vi "PCU_Sample.vi"() -> ()   [LabVIEW 2017]
uses:
  D:/test/FULLband-sts/Fullband_Sample/DLL/InstrumentDLL.dll
  DLL/InstrumentDLL.dll
panel:
  out "PCU":refnum<k24>
  out "LAN Port number":i32
  in  "Btn_GetLAN_Port":bool
  out "IP Address":string
  in  "Btn_GetIPAddress":bool
  in  "btnGet_Range":bool
  out "txtcurrentrange":string
  in  "btnAdjust_Range":bool
  in  "btnSet_SOP":bool
  in  "SOP Stauts":u16(ring)
  out "Serial number":string
  out "Product":string
  out "F/ W Vesion":string
  out "Wavelength range":string
  out "PCU-100 Control ID":string
  in  "Port number":i32
  in  "Target":enum32{"rdo100", "rdo110"}(radio)
  in  "Communication":T1(radio)
  in  "Terminator":enum32{"Cr", "Lf", "CrLf"}(radio)
  in  "Btn_Connect":bool
  in  "Btn_DisConnect":bool
  in  "Address/Device number":string
  in  "btnControl_ID":bool
  in  "PCU-100 Control ID":enum16{""}(ring)
  in  "Usb resouce":enum16{""}(ring)
  in  "btnUsb_resouce":bool
  in  "USB device number":string
  in  "btnSplit":bool
  out "GPIB Address":dbl
  out "GPIB Boad":dbl
  in  "btnGet_Visa":bool
  in  "Visa String":u16(ring) items=["GPIB0::5::INSTR"]
  # "0. Connect Tool"
  # "1. Connect"
  # "Information"
  # "2.Function"
  # "Power Control"
  # "SOP Control"
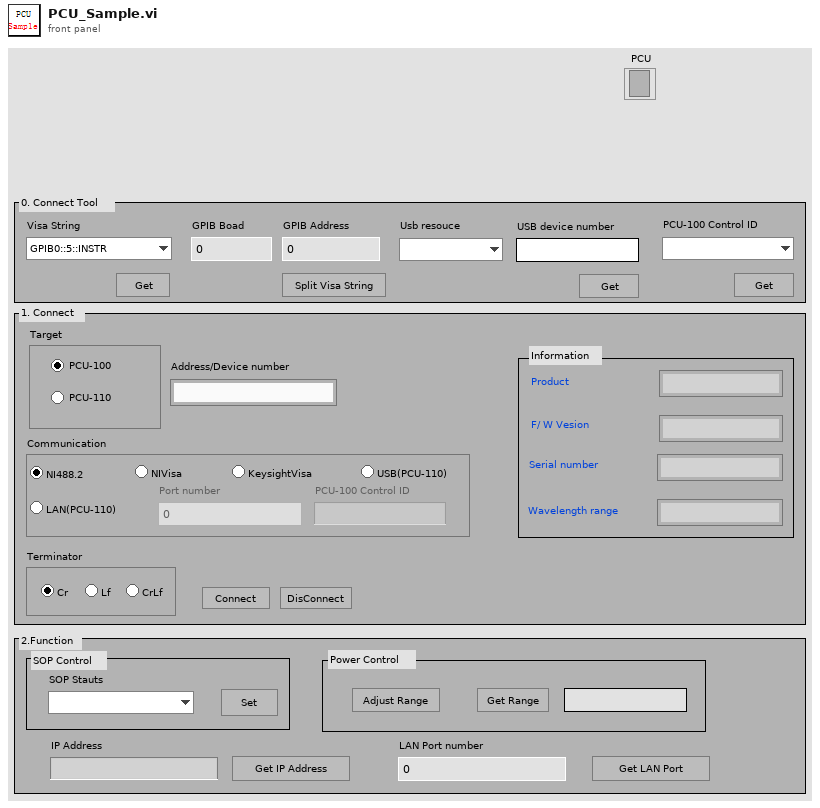
[diagram p1: front panel]
types:
  T1 = enum32{"rdiNI488", "rdiNIvisa", "rdikeysightvisa", "rdiUSB", "rdiLAN"}
  T2 = enum8{"Enabled", "Disabled", "Disabled and Grayed Out"}
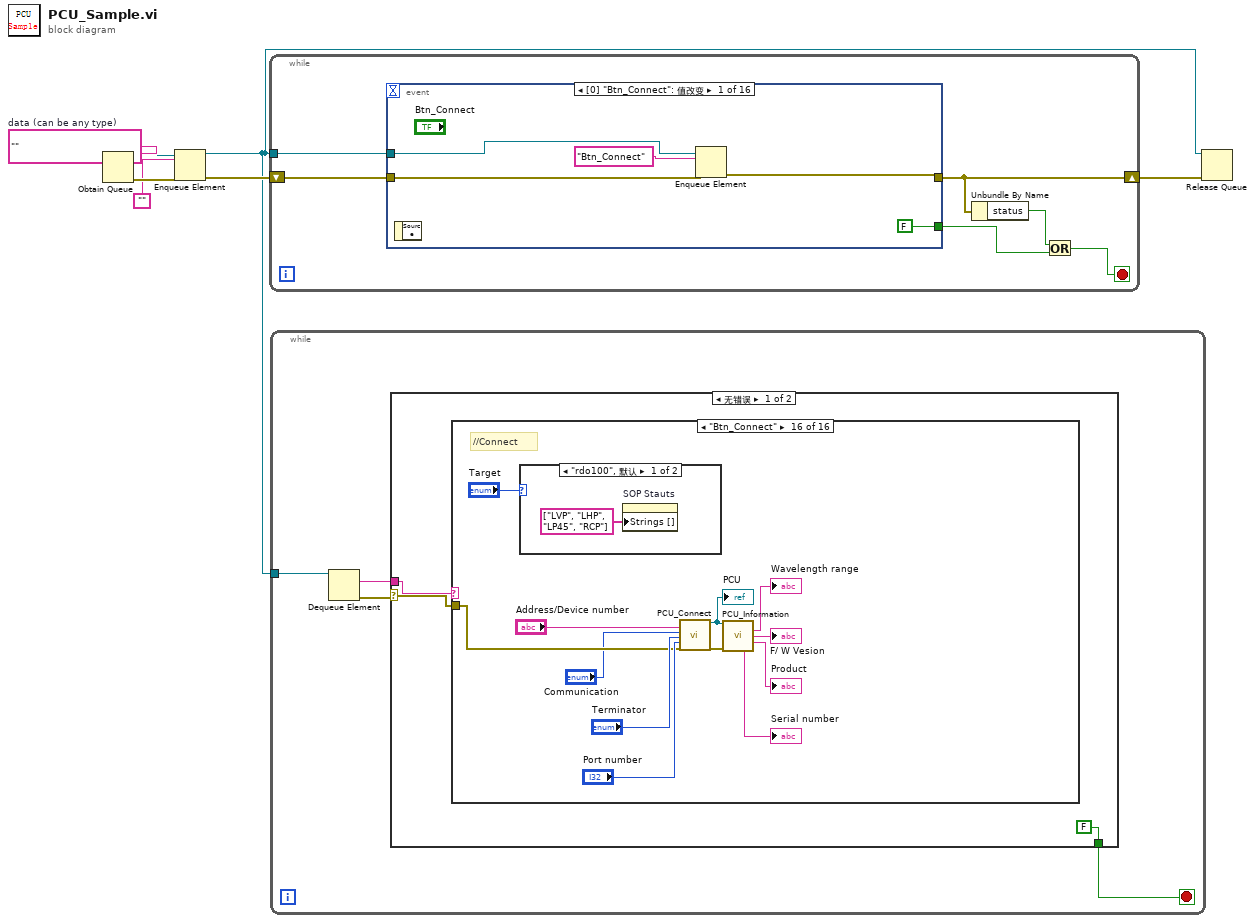
[diagram p0: block diagram]
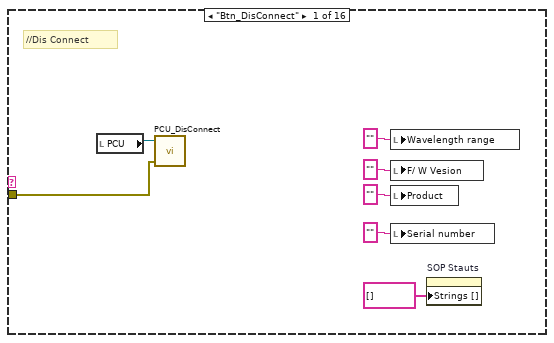
[diagram p2: hidden frame]
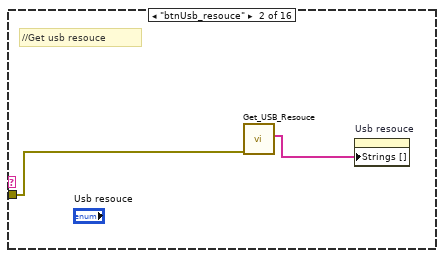
[diagram p3: hidden frame]
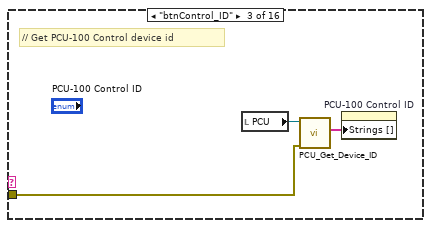
[diagram p4: hidden frame]
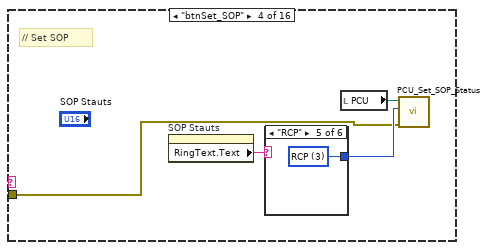
[diagram p5: hidden frame]
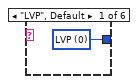
[diagram p6: hidden frame]
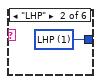
[diagram p7: hidden frame]
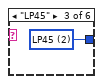
[diagram p8: hidden frame]
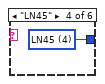
[diagram p9: hidden frame]
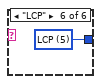
[diagram p10: hidden frame]
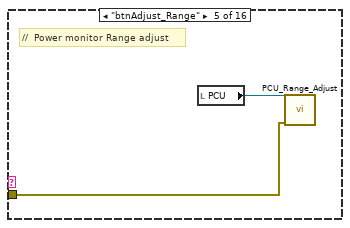
[diagram p11: hidden frame]
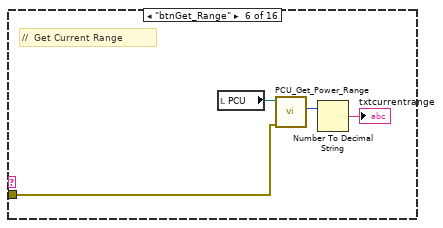
[diagram p12: hidden frame]
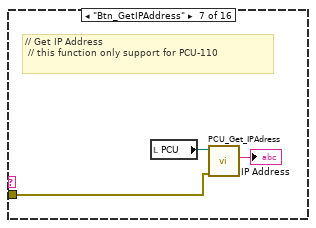
[diagram p13: hidden frame]
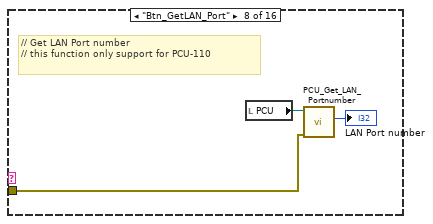
[diagram p14: hidden frame]
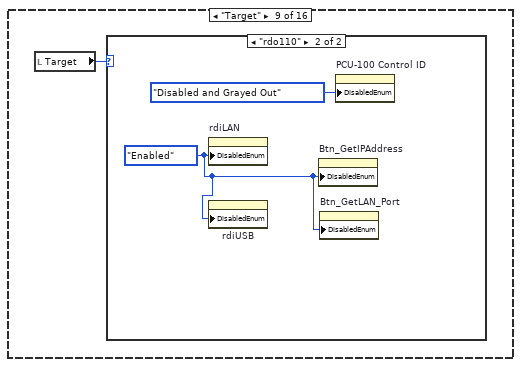
[diagram p15: hidden frame]
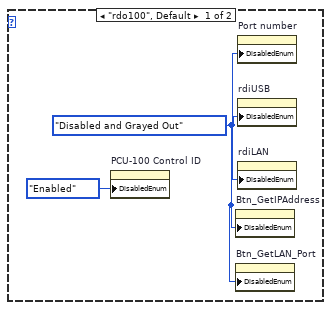
[diagram p16: hidden frame]
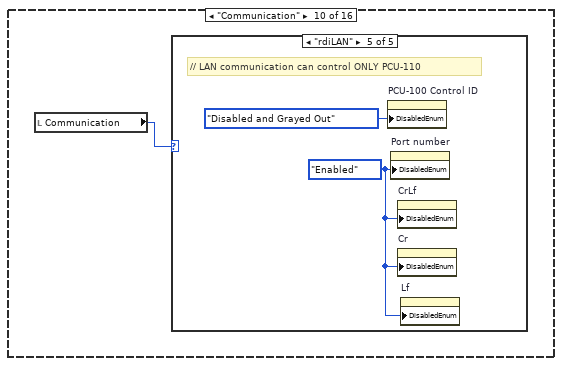
[diagram p17: hidden frame]
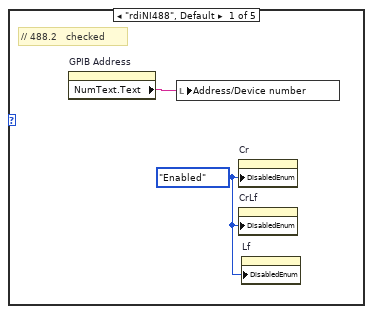
[diagram p18: hidden frame]
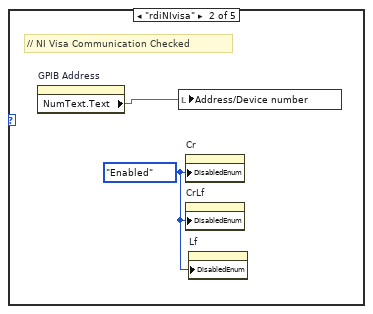
[diagram p19: hidden frame]
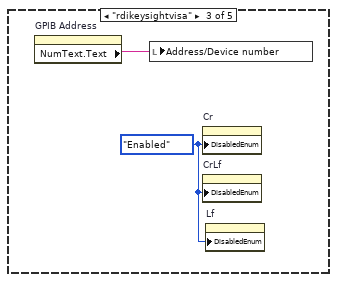
[diagram p20: hidden frame]
diagram:
  w6 = ""  # data (can be any type)
  n1 = Obtain Queue(element data type=w6) -> (queue out=w5:refnum<queue>, error out=w7:errorcluster)  [unwired: 4 in, 1 out]
  n2 = Enqueue Element(queue=w5, element="", error in (no error)=w7) -> (queue out=w1:refnum<queue>, error out=w3:errorcluster)  [unwired: 1 in, 1 out]
  n3 = while {
    tunnel: w1 -> [w12]
    shift-right: [w9] -> w2
    shift-left: w3 -> [w13]
    stop <- w10 stop-if-true
    n4 = event shown="[0] \"Btn_Connect\": 值改变" {
      selector: _ -> [_ _ _ _ _ _ _ _ _ _ _ _ _ _ _ _]
      dyn-events: _ -> [_ _ _ _ _ _ _ _ _ _ _ _ _ _ _ _]
      timeout: _ -> [_ _ _ _ _ _ _ _ _ _ _ _ _ _ _ _]
      tunnel: w13 -> [w16 w21 w26 w30 w34 w38 w42 w46 w50 w54 w58 w62 w66 w70 w74 _]
      tunnel: w12 -> [w17 w22 w25 w29 w33 w37 w41 w45 w49 w53 w57 w61 w65 w69 w73 _]
      tunnel: [w15 w20 w24 w28 w32 w36 w40 w44 w48 w52 w56 w60 w64 w68 w72 _] -> w9
      tunnel: [FALSE ("stop") FALSE ("stop") _ _ _ _ _ _ _ _ _ _ _ _ _ TRUE ("stop")] -> w8
      event "Btn_Connect": Value Change {
        n5 = event-data() -> ()  [unwired: 1 in, 1 out]
        n6 = Enqueue Element(queue=w17, element="Btn_Connect" ("元素"), error in (no error)=w16) -> (error out=w15:errorcluster)  [unwired: 1 in, 2 out]
      }
      event "Btn_DisConnect": Value Change {
        n7 = event-data() -> ()  [unwired: 1 in, 1 out]
        n8 = Enqueue Element(queue=w22, element="Btn_DisConnect" ("元素"), error in (no error)=w21) -> (error out=w20:errorcluster)  [unwired: 1 in, 2 out]
      }
      event "btnGet_Visa": Value Change {
        n9 = event-data() -> ()  [unwired: 1 in, 1 out]
        n10 = Enqueue Element(queue=w25, element="btnGet_Visa" ("元素"), error in (no error)=w26) -> (error out=w24:errorcluster)  [unwired: 1 in, 2 out]
      }
      event "btnSplit": Value Change {
        n11 = event-data() -> ()  [unwired: 1 in, 1 out]
        n12 = Enqueue Element(queue=w29, element="btnSplit" ("元素"), error in (no error)=w30) -> (error out=w28:errorcluster)  [unwired: 1 in, 2 out]
      }
      event "btnUsb_resouce": Value Change {
        n13 = event-data() -> ()  [unwired: 1 in, 1 out]
        n14 = Enqueue Element(queue=w33, element="btnUsb_resouce" ("元素"), error in (no error)=w34) -> (error out=w32:errorcluster)  [unwired: 1 in, 2 out]
      }
      event "btnControl_ID": Value Change {
        n15 = event-data() -> ()  [unwired: 1 in, 1 out]
        n16 = Enqueue Element(queue=w37, element="btnControl_ID" ("元素"), error in (no error)=w38) -> (error out=w36:errorcluster)  [unwired: 1 in, 2 out]
      }
      event "btnSet_SOP": Value Change {
        n17 = event-data() -> ()  [unwired: 1 in, 1 out]
        n18 = Enqueue Element(queue=w41, element="btnSet_SOP" ("元素"), error in (no error)=w42) -> (error out=w40:errorcluster)  [unwired: 1 in, 2 out]
      }
      event "btnAdjust_Range": Value Change {
        n19 = event-data() -> ()  [unwired: 1 in, 1 out]
        n20 = Enqueue Element(queue=w45, element="btnAdjust_Range" ("元素"), error in (no error)=w46) -> (error out=w44:errorcluster)  [unwired: 1 in, 2 out]
      }
      event "btnGet_Range": Value Change {
        n21 = event-data() -> ()  [unwired: 1 in, 1 out]
        n22 = Enqueue Element(queue=w49, element="btnGet_Range" ("元素"), error in (no error)=w50) -> (error out=w48:errorcluster)  [unwired: 1 in, 2 out]
      }
      event "Btn_GetIPAddress": Value Change {
        n23 = event-data() -> ()  [unwired: 1 in, 1 out]
        n24 = Enqueue Element(queue=w53, element="Btn_GetIPAddress" ("元素"), error in (no error)=w54) -> (error out=w52:errorcluster)  [unwired: 1 in, 2 out]
      }
      event "Btn_GetLAN_Port": Value Change {
        n25 = event-data() -> ()  [unwired: 1 in, 1 out]
        n26 = Enqueue Element(queue=w57, element="Btn_GetLAN_Port" ("元素"), error in (no error)=w58) -> (error out=w56:errorcluster)  [unwired: 1 in, 2 out]
      }
      event "Target": Value Change {
        n27 = event-data() -> ()  [unwired: 1 in, 1 out]
        n28 = Enqueue Element(queue=w61, element="Target" ("元素"), error in (no error)=w62) -> (error out=w60:errorcluster)  [unwired: 1 in, 2 out]
      }
      event "Communication": Value Change {
        n29 = event-data() -> ()  [unwired: 1 in, 1 out]
        n30 = Enqueue Element(queue=w65, element="Communication" ("元素"), error in (no error)=w66) -> (error out=w64:errorcluster)  [unwired: 1 in, 2 out]
      }
      event "Usb resouce": Value Change {
        n31 = event-data() -> ()  [unwired: 1 in, 1 out]
        n32 = Enqueue Element(queue=w69, element="Usb resouce" ("元素"), error in (no error)=w70) -> (error out=w68:errorcluster)  [unwired: 1 in, 2 out]
      }
      event "PCU-100 Control ID": Value Change {
        n33 = event-data() -> ()  [unwired: 1 in, 1 out]
        n34 = Enqueue Element(queue=w73, element="PCU-100 Control ID" ("元素"), error in (no error)=w74) -> (error out=w72:errorcluster)  [unwired: 1 in, 2 out]
      }
      event Panel Close {
        n35 = event-data() -> ()  [unwired: 1 in, 1 out]
      }
    }
    n36 = Unbundle By Name(w9) -> ("status"=w11:bool)
    n37 = Or(x=w11, y=w8) -> (x .or. y?=w10:bool)
  }
  n38 = while {
    tunnel: w1 -> [w79]
    stop <- w77 stop-if-true
    n39 = Dequeue Element(queue=w79) -> (element=w78:string, error out=w80:errorcluster)  [unwired: 2 in, 2 out]
    n40 = case shown="无错误" w80 {
      selector: w80 -> [w81 _]
      tunnel: w78 -> [w83 _]
      tunnel: [FALSE TRUE] -> w77
      frame No Error {
        n41 = case shown="\"Btn_Connect\"" w83 {
          tunnel: w81 -> [w84 w91 w93 w96 w106 w108 w112 w115 _ _ _ _ _ w139 _ w163]
          frame "Btn_DisConnect" {
            # "//Dis Connect"
            n42 = local read "PCU"() -> (w85:refnum<k24>)
            n43 = call "PCU_DisConnect.vi"("error in (no error)"=w84, ".NET Reference in"=w85) -> ()  [unwired: 2 in, 2 out]
            n44 = local write "Wavelength range"("" ("Wavelength range")) -> ()
            n45 = local write "F/ W Vesion"("" ("F/ W Vesion")) -> ()
            n46 = local write "Product"("" ("Product")) -> ()
            n47 = local write "Serial number"("" ("Serial number")) -> ()
            n48 = property on="SOP Stauts" class="Ring (严格)"("Strings []"=string[] [] ("字符串[]")) -> ()  [unwired: 2 in, 2 out]
          }
          frame "btnUsb_resouce" {
            # "//Get usb resouce"
            n49 = call "Get_USB_Resouce.vi"("error in (no error)"=w91) -> ("Get_USB_Resouce"=w92:string[])  [unwired: 8 in, 2 out]
            n50 = property on="Usb resouce" class="Enum (严格)"("Strings []"=w92) -> ()  [unwired: 2 in, 2 out]
          }
          frame "btnControl_ID" {
            # "// Get PCU-100 Control device id"
            n51 = local read "PCU"() -> (w95:refnum<k24>)
            n52 = call "PCU_Get_Device_ID.vi"("error in (no error)"=w93, ".NET Reference in"=w95) -> ("id"=w94:string[])  [unwired: 7 in, 2 out]
            n53 = property on="PCU-100 Control ID" class="Enum (严格)"("Strings []"=w94) -> ()  [unwired: 2 in, 2 out]
          }
          frame "btnSet_SOP" {
            # "// Set SOP"
            n54 = property on="SOP Stauts" class="Ring (严格)"() -> ("RingText.Text"=w98:string)  [unwired: 2 in, 2 out]
            n55 = case shown="\"RCP\"" w98 {
              tunnel: [w100 w101 w102 w103 w104 w105] -> w97
              frame "LVP", Default {
                w100 = 0 items=["LVP", "LHP", "LP45", "RCP", "LN45", "LCP"] ("status")
              }
              frame "LHP" {
                w101 = 1 items=["LVP", "LHP", "LP45", "RCP", "LN45", "LCP"] ("status")
              }
              frame "LP45" {
                w102 = 2 items=["LVP", "LHP", "LP45", "RCP", "LN45", "LCP"] ("status")
              }
              frame "LN45" {
                w103 = 4 items=["LVP", "LHP", "LP45", "RCP", "LN45", "LCP"] ("status")
              }
              frame "RCP" {
                w104 = 3 items=["LVP", "LHP", "LP45", "RCP", "LN45", "LCP"] ("status")
              }
              frame "LCP" {
                w105 = 5 items=["LVP", "LHP", "LP45", "RCP", "LN45", "LCP"] ("status")
              }
            }
            n56 = local read "PCU"() -> (w99:refnum<k24>)
            n57 = call "PCU_Set_SOP_Status.vi"("error in (no error)"=w96, "status"=w97, ".NET Reference in"=w99) -> ()  [unwired: 7 in, 2 out]
          }
          frame "btnAdjust_Range" {
            # "//  Power monitor Range adjust"
            n58 = local read "PCU"() -> (w107:refnum<k24>)
            n59 = call "PCU_Range_Adjust.vi"("error in (no error)"=w106, ".NET Reference in"=w107) -> ()  [unwired: 8 in, 2 out]
          }
          frame "btnGet_Range" {
            # "//  Get Current Range"
            n60 = local read "PCU"() -> (w111:refnum<k24>)
            n61 = call "PCU_Get_Power_Range.vi"("error in (no error)"=w108, ".NET Reference in"=w111) -> ("range"=w109:i32)  [unwired: 7 in, 2 out]
            n62 = Number To Decimal String(number=w109) -> (decimal integer string=→"txtcurrentrange":string)  [unwired: 1 in]
          }
          frame "Btn_GetIPAddress" {
            # "// Get IP Address\n // this function only support for PCU-110"
            n63 = local read "PCU"() -> (w114:refnum<k24>)
            n64 = call "PCU_Get_IPAdress.vi"("error in (no error)"=w112, ".NET Reference in"=w114) -> ("address"=→"IP Address":string)  [unwired: 7 in, 2 out]
          }
          frame "Btn_GetLAN_Port" {
            # "// Get LAN Port number\n// this function only support for PCU-110"
            n65 = local read "PCU"() -> (w117:refnum<k24>)
            n66 = call "PCU_Get_LAN_Portnumber.vi"("error in (no error)"=w115, ".NET Reference in"=w117) -> ("port"=→"LAN Port number":i32)  [unwired: 7 in, 2 out]
          }
          frame "Target" {
            n67 = local read "Target"() -> (w118:enum32{"rdo100", "rdo110"})
            n68 = case shown="\"rdo110\"" w118 {
              frame "rdo100", Default {
                w119 = T2."Disabled and Grayed Out" ("禁用")
                n69 = property on="PCU-100 Control ID" class="Str"("DisabledEnum"=T2."Enabled" ("禁用")) -> ()  [unwired: 2 in, 2 out]
                n70 = property on="Btn_GetIPAddress" class="Bool"("DisabledEnum"=w119) -> ()  [unwired: 2 in, 2 out]
                n71 = property on="Btn_GetLAN_Port" class="Bool"("DisabledEnum"=w119) -> ()  [unwired: 2 in, 2 out]
                n72 = property on="Port number" class="DigNum (严格)"("DisabledEnum"=w119) -> ()  [unwired: 2 in, 2 out]
                n73 = property on="rdiUSB" class="Bool (严格)"("DisabledEnum"=w119) -> ()  [unwired: 2 in, 2 out]
                n74 = property on="rdiLAN" class="Bool (严格)"("DisabledEnum"=w119) -> ()  [unwired: 2 in, 2 out]
              }
              frame "rdo110" {
                w121 = T2."Enabled" ("禁用")
                n75 = property on="rdiLAN" class="Bool (严格)"("DisabledEnum"=w121) -> ()  [unwired: 2 in, 2 out]
                n76 = property on="rdiUSB" class="Bool (严格)"("DisabledEnum"=w121) -> ()  [unwired: 2 in, 2 out]
                n77 = property on="Btn_GetIPAddress" class="Bool"("DisabledEnum"=w121) -> ()  [unwired: 2 in, 2 out]
                n78 = property on="Btn_GetLAN_Port" class="Bool"("DisabledEnum"=w121) -> ()  [unwired: 2 in, 2 out]
                n79 = property on="PCU-100 Control ID" class="Str"("DisabledEnum"=T2."Disabled and Grayed Out" ("禁用")) -> ()  [unwired: 2 in, 2 out]
              }
            }
          }
          frame "Communication" {
            n80 = local read "Communication"() -> (w123:T1)
            n81 = case shown="\"rdiLAN\"" w123 {
              frame "rdiNI488", Default {
                w125 = T2."Enabled" ("禁用")
                # "// 488.2　checked"
                n82 = property on="GPIB Address" class="DigNum (严格)"() -> ("NumText.Text"=w124:string)  [unwired: 2 in, 2 out]
                n83 = local write "Address/Device number"(w124) -> ()
                n84 = property on="Cr" class="Bool (严格)"("DisabledEnum"=w125) -> ()  [unwired: 2 in, 2 out]
                n85 = property on="CrLf" class="Bool (严格)"("DisabledEnum"=w125) -> ()  [unwired: 2 in, 2 out]
                n86 = property on="Lf" class="Bool (严格)"("DisabledEnum"=w125) -> ()  [unwired: 2 in, 2 out]
              }
              frame "rdiNIvisa" {
                w127 = T2."Enabled" ("禁用")
                # "// NI Visa Communication Checked"
                n87 = property on="GPIB Address" class="DigNum (严格)"() -> ("NumText.Text"=w126:string)  [unwired: 2 in, 2 out]
                n88 = local write "Address/Device number"(w126) -> ()
                n89 = property on="Cr" class="Bool (严格)"("DisabledEnum"=w127) -> ()  [unwired: 2 in, 2 out]
                n90 = property on="CrLf" class="Bool (严格)"("DisabledEnum"=w127) -> ()  [unwired: 2 in, 2 out]
                n91 = property on="Lf" class="Bool (严格)"("DisabledEnum"=w127) -> ()  [unwired: 2 in, 2 out]
              }
              frame "rdikeysightvisa" {
                w129 = T2."Enabled" ("禁用")
                n92 = property on="GPIB Address" class="DigNum (严格)"() -> ("NumText.Text"=w128:string)  [unwired: 2 in, 2 out]
                n93 = local write "Address/Device number"(w128) -> ()
                n94 = property on="Cr" class="Bool (严格)"("DisabledEnum"=w129) -> ()  [unwired: 2 in, 2 out]
                n95 = property on="CrLf" class="Bool (严格)"("DisabledEnum"=w129) -> ()  [unwired: 2 in, 2 out]
                n96 = property on="Lf" class="Bool (严格)"("DisabledEnum"=w129) -> ()  [unwired: 2 in, 2 out]
              }
              frame "rdiUSB" {
                w131 = T2."Disabled and Grayed Out" ("禁用")
                # "// USB can control Only PCU-110"
                n97 = local write "Address/Device number"("USB device number") -> ()
                n98 = property on="Cr" class="Bool (严格)"("Key Focus"=TRUE ("键选中")) -> ()  [unwired: 2 in, 2 out]
                n99 = property on="CrLf" class="Bool (严格)"("DisabledEnum"=w131) -> ()  [unwired: 2 in, 2 out]
                n100 = property on="Lf" class="Bool (严格)"("DisabledEnum"=w131) -> ()  [unwired: 2 in, 2 out]
              }
              frame "rdiLAN" {
                w133 = T2."Enabled" ("禁用")
                # "// LAN communication can control ONLY PCU-110"
                n101 = property on="PCU-100 Control ID" class="Str"("DisabledEnum"=T2."Disabled and Grayed Out" ("禁用")) -> ()  [unwired: 2 in, 2 out]
                n102 = property on="Port number" class="DigNum (严格)"("DisabledEnum"=w133) -> ()  [unwired: 2 in, 2 out]
                n103 = property on="CrLf" class="Bool (严格)"("DisabledEnum"=w133) -> ()  [unwired: 2 in, 2 out]
                n104 = property on="Cr" class="Bool (严格)"("DisabledEnum"=w133) -> ()  [unwired: 2 in, 2 out]
                n105 = property on="Lf" class="Bool (严格)"("DisabledEnum"=w133) -> ()  [unwired: 2 in, 2 out]
              }
            }
          }
          frame "Usb resouce" {
            # "// Select usb  resouce & Show deveice number"
            n106 = property on="Usb resouce" class="Enum (严格)"() -> ("RingText.Text"=w135:string)  [unwired: 2 in, 2 out]
            n107 = local write "USB device number"(w135) -> ()
          }
          frame "PCU-100 Control ID" {
            # "//      Select control device number for PCU-100"
            n108 = property on="PCU-100 Control ID" class="Enum (严格)"() -> ("RingText.Text"=→"PCU-100 Control ID":string)  [unwired: 2 in, 2 out]
          }
          frame "Load", Default {
            # "// ----PCU-100　check"
            n109 = property on="rdo100" class="Bool (严格)"("Key Focus"=TRUE ("键选中")) -> ()  [unwired: 2 in, 2 out]
            n110 = property on="rdo110" class="Bool (严格)"("Key Focus"=FALSE ("键选中")) -> ()  [unwired: 2 in, 2 out]
          }
          frame "btnGet_Visa" {
            # "// Get GPIB resouce"
            n111 = call "Get_GPIB_Resouces.vi"("error in (no error)"=w139) -> ("Get_GPIB_Resources"=w140:string[])  [unwired: 8 in, 2 out]
            n112 = property on="Visa String" class="Ring (严格)"("Strings []"=w140) -> ()  [unwired: 2 in, 2 out]
          }
          frame "btnSplit" {
            # "// Split visa string"
            n113 = property on="Visa String" class="Ring (严格)"() -> ("RingText.Text"=w148:string)  [unwired: 2 in, 2 out]
            n114 = while {
              shift-right: [w157] -> _
              shift-left: w148 -> [w159]
              shift-right: [w152] -> _
              shift-left: 0 ("偏移量") -> [w158]
              shift-right: [w153] -> w144
              shift-left: dbl[] [] ("数组") -> [w154]
              stop <- w150 stop-if-true
              n115 = Scan String For Tokens(6:string[] [":"] ("分隔符(\\s,\\t,\\r,\\n)"), 8:w158, 9:w159) -> (1:w156:string, 2:w152:i32, 3:w157:string)  [unwired: 3 in, 1 out]
              n116 = Fract/Exp String To Number(string=w156) -> (number=w155:dbl)  [unwired: 3 in, 1 out]
              n117 = Equal?(x=w152, y=-1) -> (x = y?=w150:bool)
              n118 = Build Array (concatenate)(w154, w155) -> (w153:dbl[])
            }
            n119 = Index Array(array=w144, index=0 ("索引")) -> (element=→"GPIB Boad":dbl)
            n120 = Index Array(array=w144, index=1 ("索引")) -> (element=→"GPIB Address":dbl)
          }
          frame "Btn_Connect" {
            # "//Connect"
            n121 = case shown="\"rdo100\", 默认" "Target" {
              frame "rdo100", Default {
                n122 = property on="SOP Stauts" class="Ring (严格)"("Strings []"=string[] ["LVP", "LHP", "LP45", "RCP"] ("字符串[]")) -> ()  [unwired: 2 in, 2 out]
              }
              frame "rdo110" {
                n123 = property on="SOP Stauts" class="Ring (严格)"("Strings []"=string[] ["LVP", "LHP", "LP45", "LN45", "RCP", "LCP"] ("字符串[]")) -> ()  [unwired: 2 in, 2 out]
              }
            }
            n124 = call "PCU_Connect.vi"("Address/ComPort"="Address/Device number", "Communication"="Communication", "Terminator"="Terminator", "Portnumber"="Port number", "error in"=w163) -> ("Reference out"=w162:refnum<k24>, "error out"=w161:errorcluster)  [unwired: 13 in]
            "PCU" <- w162
            n125 = call "PCU_Information.vi"(".NET Reference in"=w162, "error in (no error)"=w161) -> ("Band"=→"Wavelength range":string, "FWversion"=→"F/ W Vesion":string, "ProductName"=→"Product":string, "SerialNumber"=→"Serial number":string)  [unwired: 8 in, 2 out]
          }
        }
      }
      frame Error {
      }
    }
  }
  n126 = Release Queue(queue=w1, error in (no error)=w2) -> ()  [unwired: 1 in, 3 out]
